vi "Write B-Scan Info Array.vi"(8 "error in (no error)":errorcluster, 10 "B-Scan Info Array":T1[](array[typedef]), 11 "Read in":refnum<class "Read.lvclass">) -> (0 "error out":errorcluster, 3 "Read out":refnum<class "Read.lvclass">)   [LabVIEW 2014, in "Read.lvclass"]
uses:
  Read.lvclass
  BScan.ctl
  Read.lvclass/Read.ctl
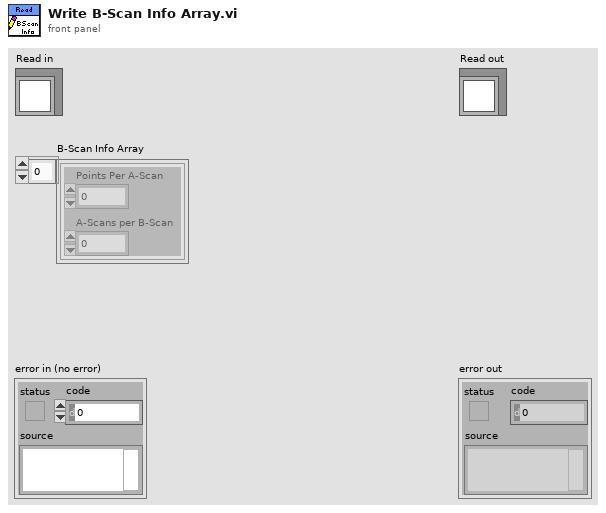
[diagram p1: front panel]
types:
  T1 = typedef "Read.lvclass/BScan.ctl" = cluster{"Points Per A-Scan":dbl, "A-Scans per B-Scan":dbl}
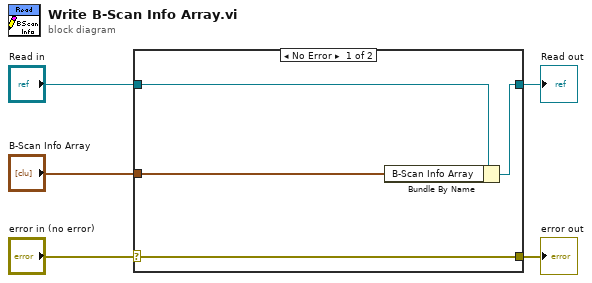
[diagram p0: block diagram]
diagram:
  n1 = case shown="No Error" "error in (no error)" {
    selector: "error in (no error)" -> [w9 w10]
    tunnel: [w9 w10] -> w4
    tunnel: [w7 w11] -> w2
    tunnel: "Read in" -> [w8 w11]
    tunnel: "B-Scan Info Array" -> [w6 _]
    frame No Error {
      n2 = Bundle By Name(cluster=w8, "B-Scan Info Array"=w6) -> (w7:refnum<class "Read.lvclass">)
    }
    frame Error {
    }
  }
  "error out" <- w4
  "Read out" <- w2
